vi "Replace Double Underscores by Parentheses.vi"(2 "String in":string) -> (7 "String out":string)   [LabVIEW 2021, in "Strings.lvlib"]
doc: "Replaces alternating double underscores by alternating parentheses: ( or ).\n\nNote that if the input strings ends with a double underscore, the output string will end with a space, and therefore some trimming might be necessary for some purposes."
uses:
  Strings.lvlib
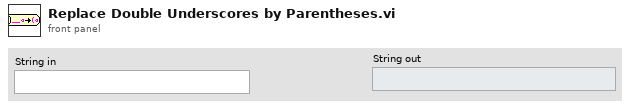
[diagram p1: front panel]
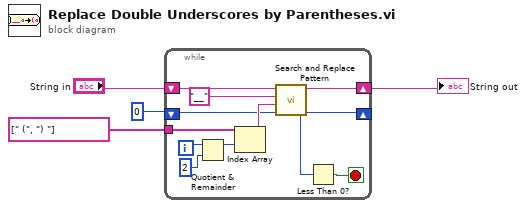
[diagram p0: block diagram]
diagram:
  n1 = while {
    shift-right: [w13] -> w3
    shift-left: "String in" -> [w15]
    tunnel: string[] [" (", ") "] ("regular expression (\"\")") -> [w10]
    shift-right: [w6] -> _
    shift-left: 0 ("offset past match") -> [w7]
    i -> [w12]
    stop <- w5 stop-if-true
    n2 = Quotient & Remainder(x=w12, y=2) -> (x-y*floor(x/y)=w9:i32)  [unwired: 1 out]
    n3 = Index Array(array=w10, index=w9) -> (element=w8:string)
    n4 = call <vilib>:"Search and Replace Pattern.vi"("string"=w15, "regular expression (\"\")"="__" ("regular expression (\"\")"), "replace string (\"\")"=w8, "offset (0)"=w7) -> ("result string"=w13:string, "offset past match"=w6:i32)  [unwired: 1 in]
    n5 = Less Than 0?(x=w6) -> (x < 0?=w5:bool)
  }
  "String out" <- w3
